vi "Reset.vi"(11 "Hash Function in":refnum<class "NI_SHA-512.lvclass">) -> (3 "Hash Function out":refnum<class "NI_SHA-512.lvclass">)   [LabVIEW 2020, in "NI_SHA-512.lvclass"]
uses:
  <vilib>/security/Message Digest/SHA-2/SHA-512/NI_SHA-512.lvclass
  <vilib>/security/Message Digest/SHA-2/SHA-512/NI_SHA-512.lvclass/NI_SHA-512.ctl
  <vilib>/security/Message Digest/SHA-2/SHA-512/subVIs/Mode.ctl
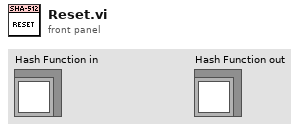
[diagram p1: front panel]
types:
  T1 = typedef "NI_SHA-512.lvclass/Mode.ctl" = enum16{"SHA-512", "SHA-384", "SHA-512/256", "SHA-512/224"}
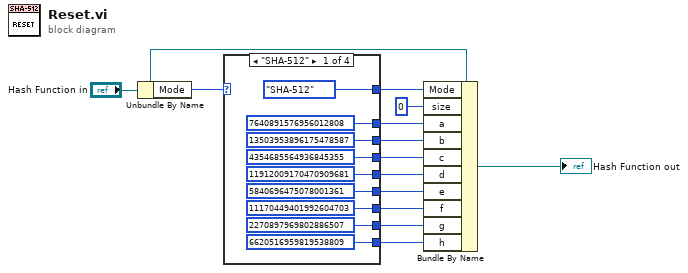
[diagram p0: block diagram]
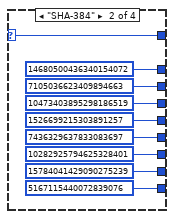
[diagram p2: hidden frame]
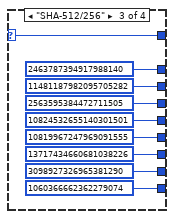
[diagram p3: hidden frame]
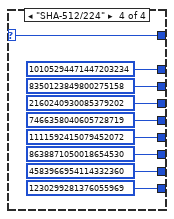
[diagram p4: hidden frame]
diagram:
  n1 = Unbundle By Name("Hash Function in") -> ("Mode"=w11:T1)
  n2 = case shown="\"SHA-512\"" w11 {
    selector: w11 -> [_ w23 w32 w41]
    tunnel: [u64 7640891576956012808 ("Numeric") u64 14680500436340154072 ("Numeric") u64 2463787394917988140 ("Numeric") u64 10105294471447203234 ("Numeric")] -> w9
    tunnel: [u64 13503953896175478587 ("Numeric") u64 7105036623409894663 ("Numeric") u64 11481187982095705282 ("Numeric") u64 8350123849800275158 ("Numeric")] -> w8
    tunnel: [u64 4354685564936845355 ("Numeric") u64 10473403895298186519 ("Numeric") u64 2563595384472711505 ("Numeric") u64 2160240930085379202 ("Numeric")] -> w7
    tunnel: [u64 11912009170470909681 ("Numeric") u64 1526699215303891257 ("Numeric") u64 10824532655140301501 ("Numeric") u64 7466358040605728719 ("Numeric")] -> w6
    tunnel: [u64 5840696475078001361 ("Numeric") u64 7436329637833083697 ("Numeric") u64 10819967247969091555 ("Numeric") u64 1111592415079452072 ("Numeric")] -> w5
    tunnel: [u64 11170449401992604703 ("Numeric") u64 10282925794625328401 ("Numeric") u64 13717434660681038226 ("Numeric") u64 8638871050018654530 ("Numeric")] -> w4
    tunnel: [u64 2270897969802886507 ("Numeric") u64 15784041429090275239 ("Numeric") u64 3098927326965381290 ("Numeric") u64 4583966954114332360 ("Numeric")] -> w3
    tunnel: [u64 6620516959819538809 ("Numeric") u64 5167115440072839076 ("Numeric") u64 1060366662362279074 ("Numeric") u64 1230299281376055969 ("Numeric")] -> w2
    tunnel: [Mode."SHA-512" ("Mode") w23 w32 w41] -> w1
    frame "SHA-512" {
    }
    frame "SHA-384" {
    }
    frame "SHA-512/256" {
    }
    frame "SHA-512/224" {
    }
  }
  n3 = Bundle By Name(cluster="Hash Function in", "Mode"=w1, "size"=u64 0, "a"=w9, "b"=w8, "c"=w7, "d"=w6, "e"=w5, "f"=w4, "g"=w3, "h"=w2) -> (→"Hash Function out":refnum<class "NI_SHA-512.lvclass">)
